vi "VIRef.vi"() -> ()   [LabVIEW 2020]
panel:
  in  "reference":refnum<vi>
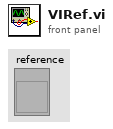
[diagram p1: front panel]
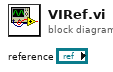
[diagram p0: block diagram]
diagram:
